vi "PKYK_Data_Format.vi"(10 "Cluster in":T2 {"MachineCode" items=["MCIG", "MCPC", "MCSA", "MCCA", "MCAC", "MCLA", "MCCM", "MCSC", "MCPA", "MCLP", "MCHP", "MCBC", "MCFA", "MCSR", "MCFV"]; "ExpiryDate" format="%<%I:%M:%S%3u %p\n%d-%m-%Y>T"; "EntDt" format="%<%I:%M:%S%3u %p\n%d-%m-%Y>T"; "UpdDt" format="%<%I:%M:%S%3u %p\n%d-%m-%Y>T"}, 11 "Pokayoke Data":variant[](array[variant])) -> (3 "Pokayoke Data Out":T2 {"MachineCode" items=["MCIG", "MCPC", "MCSA", "MCCA", "MCAC", "MCLA", "MCCM", "MCSC", "MCPA", "MCLP", "MCHP", "MCBC", "MCFA", "MCSR", "MCFV"]; "ExpiryDate" format="%<%I:%M:%S%3u %p\n%d-%m-%Y>T"; "EntDt" format="%<%I:%M:%S%3u %p\n%d-%m-%Y>T"; "UpdDt" format="%<%I:%M:%S%3u %p\n%d-%m-%Y>T"})   [LabVIEW 2020]
uses:
  Controls/Line_PKYK.ctl
  Controls/PARA_CONTROL_STR.ctl
  Controls/PKYK_MCODE.ctl
  Controls/PKYK_DATE.ctl
  Controls/PKYK_Result.ctl
panel:
  in  "ExpResult":T1=enum."PASS" caption="Expected Result"
  out "error out":errorcluster
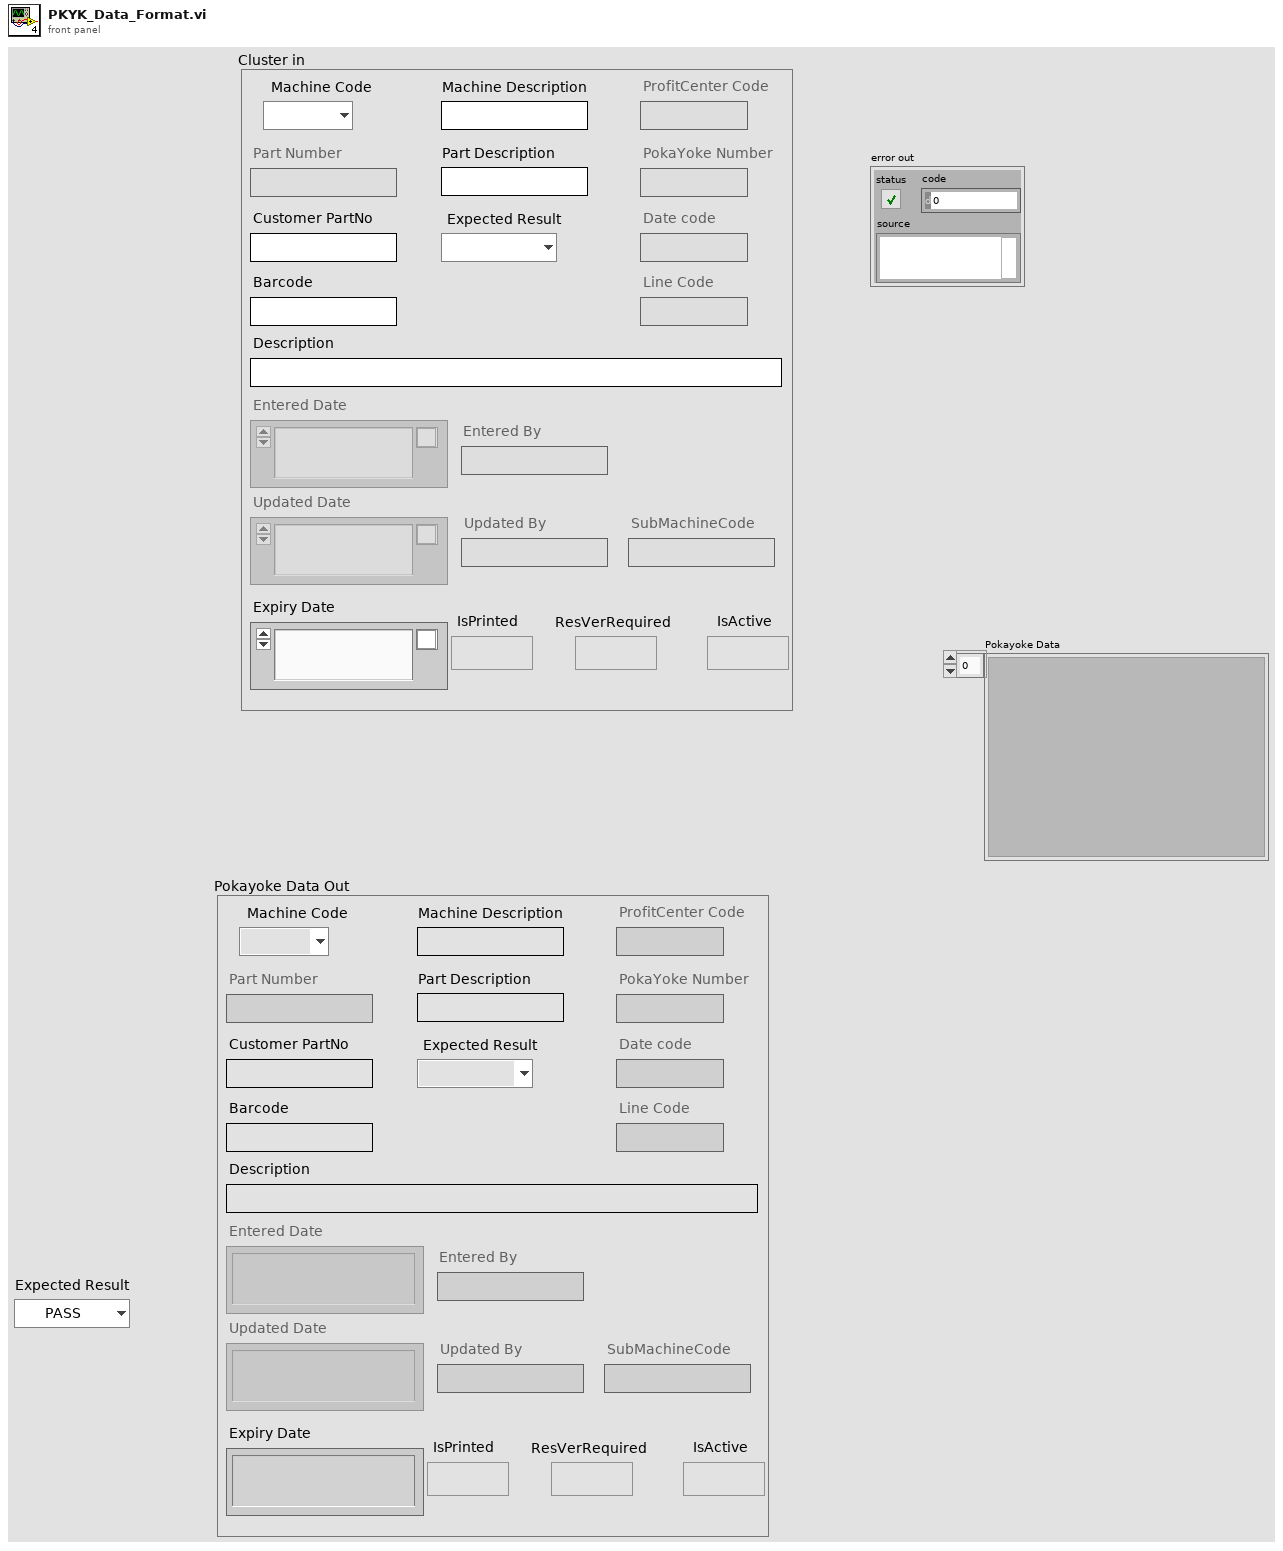
[diagram p1: front panel]
types:
  T1 = typedef "PKYK_Result.ctl" = enum16{"FAIL", "PASS"}
  T2 = typedef "Line_PKYK.ctl" = cluster{"ProfitCenterCode":string, "LineCode":string, "Datecode":string, "PartNumber":T3, "PartDescription":T3, "CustPartNo":T3, "MachineCode":T4, "MachineDescription":T3, "PokaYokeNumber":string, "Description":string, "ExpiryDate":T5, "Barcode":T3, "IsPrinted":bool, "IsActive":bool, "EntBy":T3, "EntDt":T5, "UpdBy":T3, "UpdDt":T5, "ExpResult":T1, "ResVerRequired":bool, "SubMachineCode":T3}
  T3 = typedef "PARA_CONTROL_STR.ctl" = string
  T4 = typedef "PKYK_MCODE.ctl" = u16
  T5 = typedef "PKYK_DATE.ctl" = timestamp
  T6 = enum16{"VT_EMPTY", "VT_NULL", "VT_I2", "VT_I4", "VT_R4", "VT_R8", "VT_CY", "VT_DATE", "VT_BSTR", "VT_DISPATCH", "VT_ERROR", "VT_BOOL", "VT_VARIANT", "VT_UNKNOWN", "VT_DECIMAL", "VT_15", "VT_I1", "VT_UI1", "VT_UI2", "VT_UI4", "VT_I8", "VT_UI8", "VT_INT", "VT_UINT", "VT_VOID", "VT_HRESULT", "VT_PTR", "VT_SAFEARRAY", "VT_CARRAY", "VT_USERDEFINED", "VT_LPSTR", "VT_LPWSTR"}
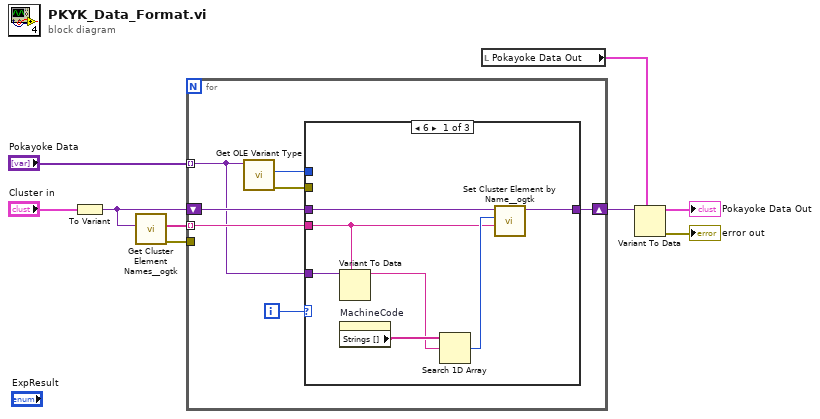
[diagram p0: block diagram]
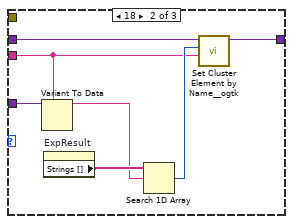
[diagram p2: hidden frame]
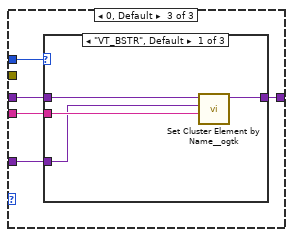
[diagram p3: hidden frame]
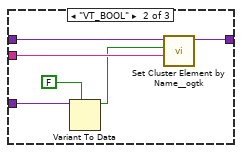
[diagram p4: hidden frame]
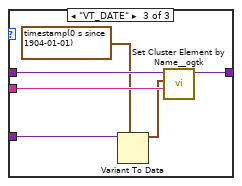
[diagram p5: hidden frame]
diagram:
  n1 = To Variant(anything="Cluster in") -> (Variant=w7:variant)
  n2 = call <userlib>:"Get Cluster Element Names__ogtk.vi"("Cluster"=w7) -> ("error out"=w1:errorcluster, "Element Names"=w8:string[])  [unwired: 9 in]
  n3 = for {
    tunnel: w8 -> [w14] mode=indexing
    shift-right: [w10] -> w4
    shift-left: w7 -> [w15]
    tunnel: "Pokayoke Data" -> [w11] mode=indexing
    tunnel: w1 -> [_]
    i -> [w16]
    n4 = call <userlib>:"Get OLE Variant Type.vi"("OLE Variant"=w11) -> ("error out"=w13:errorcluster, "variant datatype"=w12:T6)  [unwired: 3 in, 2 out]
    n5 = case shown="6" w16 {
      tunnel: w15 -> [w22 w29 w35]
      tunnel: w14 -> [w18 w25 w34]
      tunnel: [w20 w27 w33] -> w10
      tunnel: w13 -> [_ _ _]
      tunnel: w12 -> [_ _ w32]
      tunnel: w11 -> [w19 w26 w31]
      frame 6 {
        n6 = Variant To Data(type=w18, Variant=w19) -> (data=w17:string)  [unwired: 1 in, 1 out]
        n7 = property on="MachineCode" class="Ring (strict)"() -> ("Strings []"=w23:string[])  [unwired: 2 in, 2 out]
        n8 = Search 1D Array(1D array=w23, element=w17) -> (index of element=w21:i32)  [unwired: 1 in]
        n9 = call <userlib>:"Set Cluster Element by Name__ogtk.vi"("Element Name (\"\": New Element Data Name)"=w18, "New Element Value"=w21, "Cluster"=w22) -> ("VCluster out"=w20:variant)  [unwired: 6 in, 2 out]
      }
      frame 18 {
        n10 = Variant To Data(type=w25, Variant=w26) -> (data=w24:string)  [unwired: 1 in, 1 out]
        n11 = property on="ExpResult" class="Enum (strict)"() -> ("Strings []"=w30:string[])  [unwired: 2 in, 2 out]
        n12 = Search 1D Array(1D array=w30, element=w24) -> (index of element=w28:i32)  [unwired: 1 in]
        n13 = call <userlib>:"Set Cluster Element by Name__ogtk.vi"("Element Name (\"\": New Element Data Name)"=w25, "New Element Value"=w28, "Cluster"=w29) -> ("VCluster out"=w27:variant)  [unwired: 6 in, 2 out]
      }
      frame 0, Default {
        n14 = case shown="\"VT_BSTR\", Default" w32 {
          tunnel: w35 -> [w39 w45 w51]
          tunnel: w34 -> [w38 w44 w50]
          tunnel: [w37 w43 w49] -> w33
          tunnel: w31 -> [w36 w41 w48]
          frame "VT_BSTR", Default {
            n15 = call <userlib>:"Set Cluster Element by Name__ogtk.vi"("Element Name (\"\": New Element Data Name)"=w38, "New Element Value"=w36, "Cluster"=w39) -> ("VCluster out"=w37:variant)  [unwired: 6 in, 2 out]
          }
          frame "VT_BOOL" {
            n16 = Variant To Data(type=FALSE, Variant=w41) -> (data=w40:bool)  [unwired: 1 in, 1 out]
            n17 = call <userlib>:"Set Cluster Element by Name__ogtk.vi"("Element Name (\"\": New Element Data Name)"=w44, "New Element Value"=w40, "Cluster"=w45) -> ("VCluster out"=w43:variant)  [unwired: 6 in, 2 out]
          }
          frame "VT_DATE" {
            n18 = Variant To Data(type=timestamp(0 s since 1904-01-01), Variant=w48) -> (data=w46:timestamp)  [unwired: 1 in, 1 out]
            n19 = call <userlib>:"Set Cluster Element by Name__ogtk.vi"("Element Name (\"\": New Element Data Name)"=w50, "New Element Value"=w46, "Cluster"=w51) -> ("VCluster out"=w49:variant)  [unwired: 6 in, 2 out]
          }
        }
      }
    }
  }
  n20 = local read "Pokayoke Data Out"() -> (w3:T2)
  n21 = Variant To Data(type=w3, Variant=w4) -> (data=→"Pokayoke Data Out":T2, error out=→"error out":errorcluster)  [unwired: 1 in]
